vi "c_ctre_phoenix6_platform_replay_step_timing.vi"(0 "Numeric 2":dbl) -> (20 "Numeric":i32)   [LabVIEW 2023]
uses:
  <vilib>/Rock Robotics/WPI/ThirdParty/Phoenix-LabVIEW/Controls/DriverLib.ctl
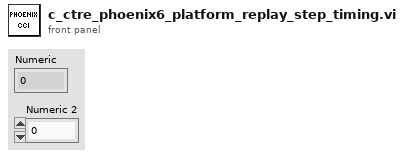
[diagram p1: front panel]
types:
  T1 = typedef "DriverLib.ctl" = path
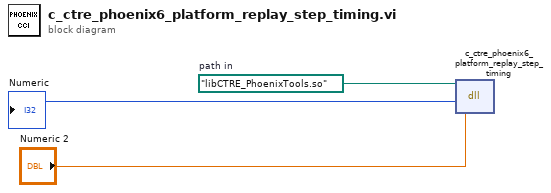
[diagram p0: block diagram]
diagram:
  w3 = T1 path "libCTRE_PhoenixTools.so"  # path in
  n1 = dll-call lib="?" fn="c_ctre_phoenix6_platform_replay_step_timing"(path in=w3, "Numeric 2") -> (→"Numeric":i32)  [unwired: 3 in, 2 out]
